vi "Parse-PNG (SubVI).vi"(11 "Unknown File":path) -> (2 "Files Found":i32, 3 "PNG Data":string[](array[string]))   [LabVIEW 2020]
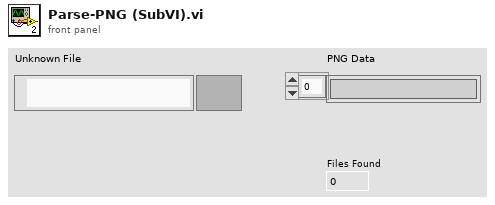
[diagram p1: front panel]
types:
  T1 = enum16{"open", "replace", "create", "open or create", "replace or create", "replace or create with confirmation"}
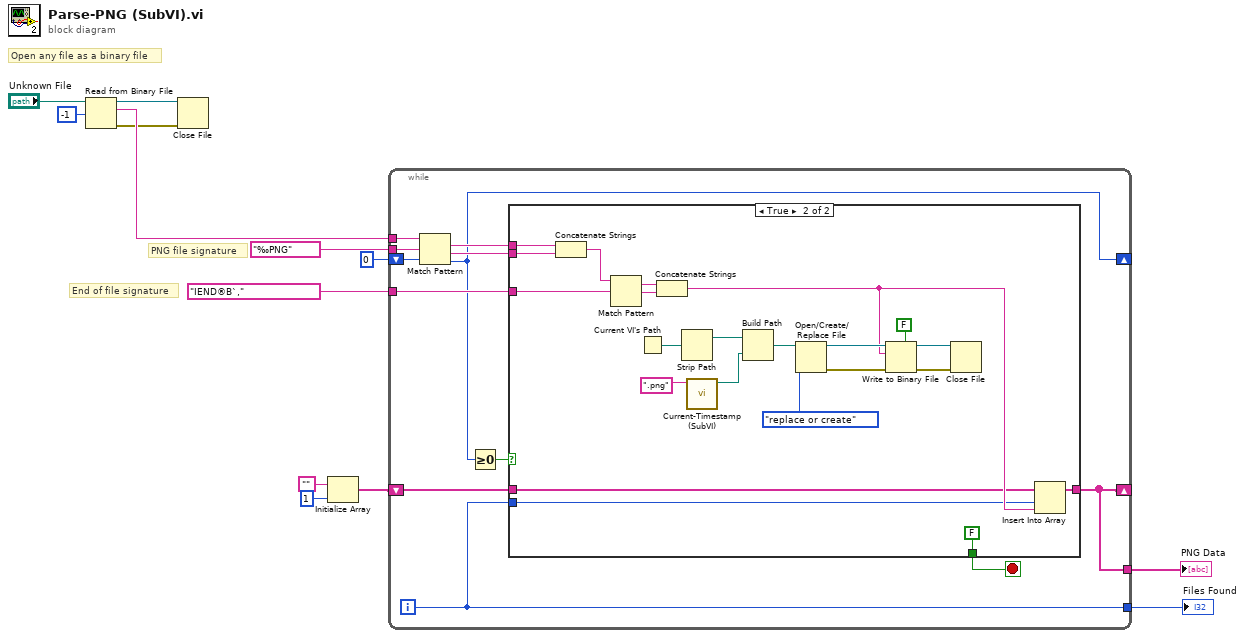
[diagram p0: block diagram]
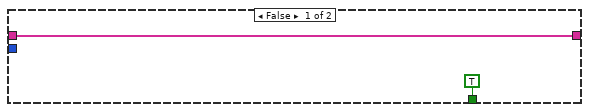
[diagram p2: hidden frame]
diagram:
  # "Open any file as a binary file"
  # "End of file signature"
  # "PNG file signature"
  n1 = Read from Binary File(10:-1 ("count (1)"), 11:"Unknown File") -> (0:w4:errorcluster, 2:w6:string, 3:w3:refnum<file>)  [unwired: 4 in, 1 out]
  n2 = Close File(refnum=w3, error in=w4) -> ()  [unwired: 2 out]
  n3 = Initialize Array("", 1 ("dimension size")) -> (w9:string[])
  n4 = while {
    tunnel: "‰PNG" -> [w21]
    tunnel: "IEND®B`‚" -> [w25]
    tunnel: w6 -> [w22]
    shift-right: [w17] -> _
    shift-left: 0 -> [w18]
    shift-right: [w15] -> _
    shift-left: w9 -> [w16]
    tunnel: [w15] -> w10
    tunnel: [w14] -> w11
    i -> [w14]
    stop <- w23 stop-if-true
    n5 = Match Pattern(string=w22, regular expression=w21, offset (0)=w18) -> (match substring=w20:string, after substring=w19:string, offset past match=w17:i32)  [unwired: 1 out]
    n6 = Greater Or Equal To 0?(x=w17) -> (x >= 0?=w24:bool)
    n7 = case shown="True" w24 {
      tunnel: w25 -> [_ w35]
      tunnel: [TRUE FALSE] -> w23
      tunnel: w20 -> [_ w33]
      tunnel: w19 -> [_ w32]
      tunnel: w16 -> [w26 w30]
      tunnel: w14 -> [_ w29]
      tunnel: [w26 w28] -> w15
      frame False {
      }
      frame True {
        n8 = Concatenate Strings(w33, w32) -> (w38:string)
        n9 = Match Pattern(string=w38, regular expression=w35) -> (before substring=w37:string, match substring=w36:string)  [unwired: 1 in, 2 out]
        n10 = Current VI's Path() -> (path=w43:path)
        n11 = Concatenate Strings(w37, w36) -> (w31:string)
        n12 = Strip Path(path=w43) -> (stripped path=w42:path)  [unwired: 1 out]
        n13 = call "Current-Timestamp (SubVI).vi"("Extension"=".png" ("string")) -> ("Path"=w49:path)  [unwired: 10 in]
        n14 = Build Path(base path=w42, name or relative path=w49) -> (appended path=w41:path)
        n15 = Open/Create/Replace File(file path (use dialog)=w41, operation (0:open)=T1."replace or create") -> (refnum out=w40:refnum<file>, error out=w46:errorcluster)  [unwired: 4 in, 1 out]
        n16 = Write to Binary File(file (use dialog)=w40, data=w31, error in=w46, 5:FALSE ("prepend array or string size? (T)")) -> (refnum out=w44:refnum<file>, error out=w45:errorcluster)  [unwired: 2 in, 1 out]
        n17 = Close File(refnum=w44, error in=w45) -> ()  [unwired: 2 out]
        n18 = Insert Into Array(array=w30, index=w29, new element=w31) -> (w28:string[])
      }
    }
  }
  "PNG Data" <- w10
  "Files Found" <- w11
